vi "Mask Write Register Request.vi"(7 "OR mask":u16, 8 "error in":errorcluster, 9 "AND mask":u16, 10 "Starting Address":u16) -> (0 "error out":errorcluster, 2 "modbus data unit out":refnum<class "Modbus Data Unit.lvclass">)   [LabVIEW 2013, in "Modbus Library - Advance.lvlib" / "Master Function Definition.lvclass"]
doc: "This VI forms a modbus data unit for masked writing of a single holding register."
uses:
  Master Function Definition.lvclass
  Modbus Data Unit/Modbus Data Unit.lvclass
  Modbus Data Unit/Function.ctl
  Modbus Data Unit/Modbus Data Unit.lvclass/Modbus Data Unit.ctl
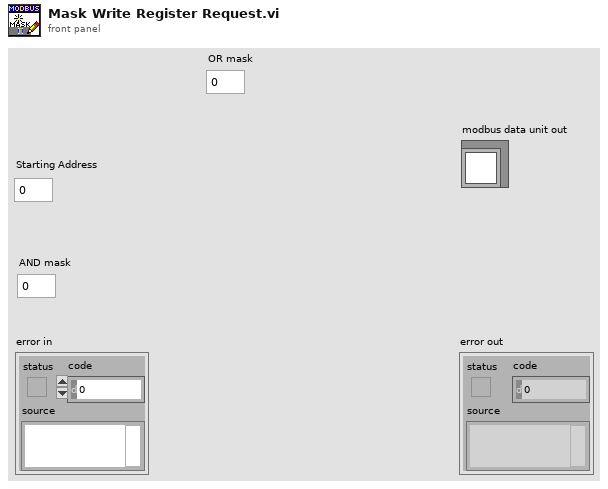
[diagram p1: front panel]
types:
  T1 = typedef "Modbus Library - Advance.lvlib/Modbus Data Unit.lvclass/Function.ctl" = u8
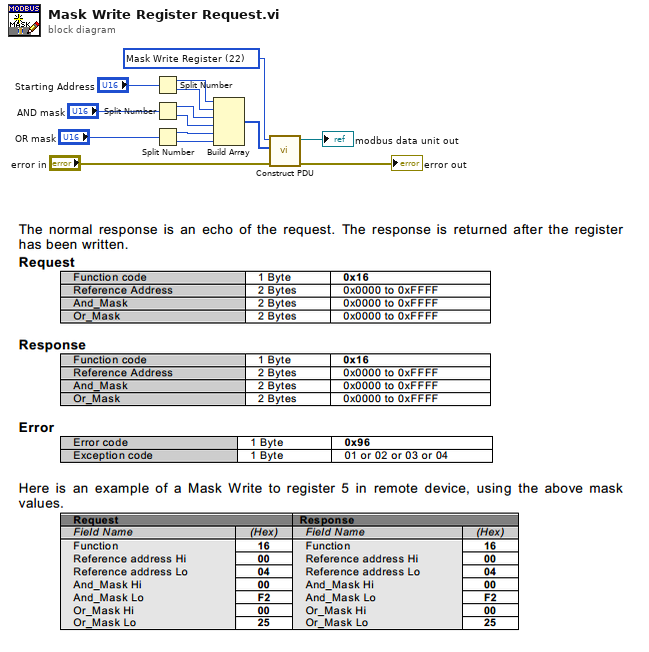
[diagram p0: block diagram]
diagram:
  w5 = T1 22 items=["Read Discrete Inputs"=2, "Read Coils"=1, "Write Single Coil"=5, "Write Multiple Coils"=15, "Read Input Register"=4, "Read Holding Registers"=3, "Write Single Register"=6, "Write Multiple Registers"=16, "Read/Write Multiple Registers"=23, "Mask Write Register"=22, "Read FIFO Queue"=24, "Read File Record"=20, "Write File Record"=21, "Read Exception Status"=7, "Diagnostic"=8, "Get Com Event Counter"=11, "Get Com Event Log"=12, "Report Slave ID"=17, "Read Device Identification"=43] ("Function")
  n1 = Split Number(x="Starting Address") -> (hi(x)=w7:u8, lo(x)=w8:u8)
  n2 = Split Number(x="AND mask") -> (hi(x)=w9:u8, lo(x)=w10:u8)
  n3 = Split Number(x="OR mask") -> (hi(x)=w1:u8, lo(x)=w2:u8)
  n4 = Build Array(w7, w8, w9, w10, w1, w2) -> (w6:u8[])
  n5 = call "Construct PDU.vi"("error in"="error in", "data"=w6, "Function"=w5) -> ("error out"=→"error out":errorcluster, "modbus data unit out"=→"modbus data unit out":refnum<class "Modbus Data Unit.lvclass">)  [unwired: 7 in]
